vi "stations.vi"(7 "httpRequestID":u32) -> ()   [LabVIEW 2011]
doc: "This VI is a state machine that can be ran from a Browser."
uses:
  server/database/Users/User Record.ctl
  <vilib>/wsapi/NI_WebServices.lvlib
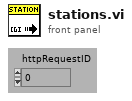
[diagram p1: front panel]
types:
  T1 = typedef "User Record.ctl" = cluster{"ixUser":i32, "sxUsername":string, "sLastName":string, "sFirstName":string, "sEmail":string, "sPassword":string, "tLoginTime":timestamp, "sLoginComputer":string, "fAdministrator":bool, "fRunSequences":bool, "fModifySequences":bool, "fRunScenarios":bool, "fModifyScenarios":bool, "fModifyTemplates":bool, "fModifyUsers":bool, "fModifyStations":bool, "fModifyFields":bool}
  T2 = typedef "Connection Refnum.ctl" = cluster{"Environment Handle":i32, "Connection Handle":i32}
  T3 = typedef "Keyed Array.ctl" = cluster{"keys":string[], "values":string[]}
  T4 = typedef "Station Record.ctl" = cluster{"ixStation":i32, "sxStationId":string, "sIP":string, "fVerified":bool}
  T5 = typedef "Instrument Record.ctl" = cluster{"ixInstrument":i32, "sxInstrumentId":string, "sDriverId":string, "sDriverType":string, "sSerialNumber":string, "tLastCalibration":timestamp, "tCalibrationDue":timestamp, "sConfiguration":string}
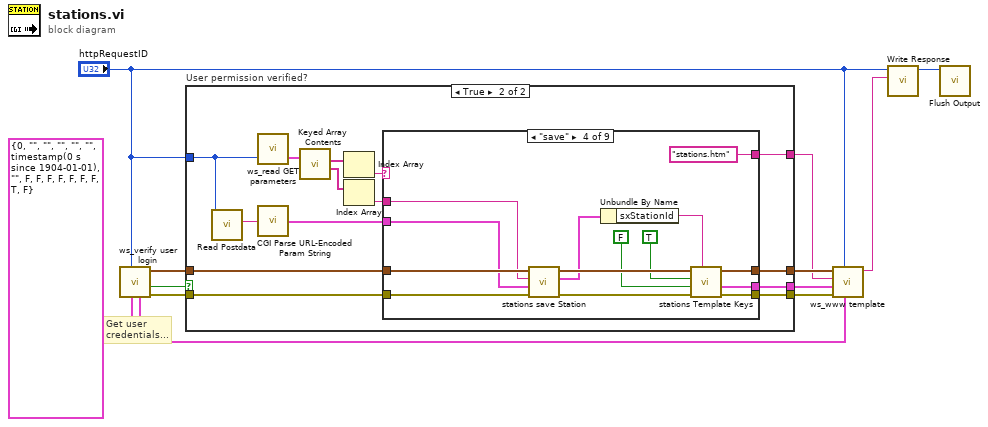
[diagram p0: block diagram]
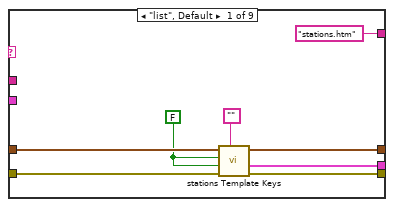
[diagram p3: hidden frame]
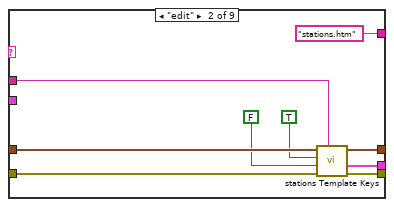
[diagram p4: hidden frame]
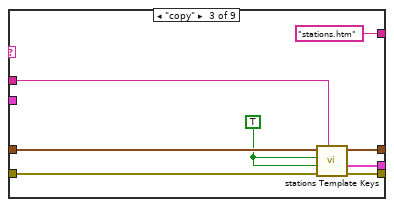
[diagram p5: hidden frame]
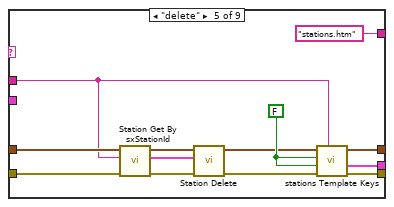
[diagram p6: hidden frame]
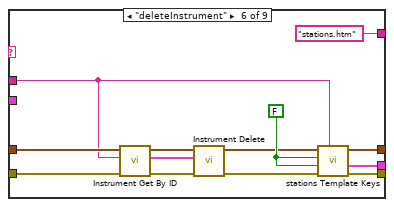
[diagram p7: hidden frame]
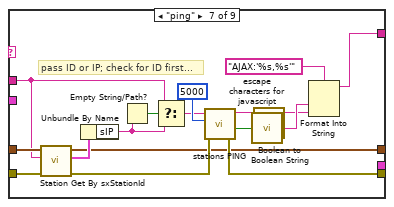
[diagram p8: hidden frame]
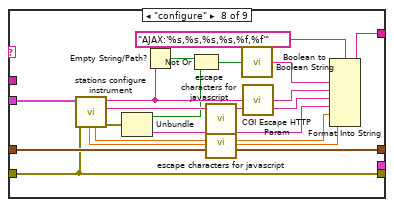
[diagram p9: hidden frame]
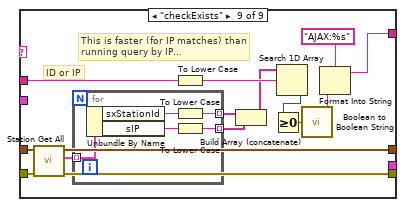
[diagram p10: hidden frame]
diagram:
  # "Get user \ncredentials..."
  n1 = call "ws_verify user login.vi"("Required Permisions"=T1 {"ixUser"=0, "sxUsername"="", "sLastName"="", "sFirstName"="", "sEmail"="", "sPassword"="", "tLoginTime"=timestamp(0 s since 1904-01-01), "sLoginComputer"="", "fAdministrator"=FALSE, "fRunSequences"=FALSE, "fModifySequences"=FALSE, "fRunScenarios"=FALSE, "fModifyScenarios"=FALSE, "fModifyTemplates"=FALSE, "fModifyUsers"=FALSE, "fModifyStations"=TRUE, "fModifyFields"=FALSE} ("User Record"), "httpRequestID"="httpRequestID") -> ("error out"=w6:errorcluster, "User Verified\nand Spartan\nAuthorized?"=w4:bool, "DB Connection Ref"=w5:T2, "User"=w3:T1)  [unwired: 6 in]
  n2 = case "User permission verified?" shown="True" w4 {
    tunnel: w5 -> [w13 w20]
    tunnel: w6 -> [w14 w21]
    tunnel: [w14 w22] -> w11
    tunnel: [_ w19] -> w9
    tunnel: [w13 w17] -> w12
    tunnel: [_ w18] -> w10
    tunnel: "httpRequestID" -> [_ w16]
    frame False {
    }
    frame True {
      n3 = call <vilib>:"Read Postdata.vi"("httpRequestID"=w16) -> ("postdata"=w15:string)  [unwired: 8 in, 2 out]
      n4 = call "ws_read GET parameters.vi"("httpRequestID"=w16) -> ("GET query params"=w23:T3)  [unwired: 2 in]
      n5 = call <vilib>:"CGI Parse URL-Encoded Param String.vi"("url-encoded param string"=w15) -> ("params"=w25:T3)
      n6 = call <vilib>:"Keyed Array Contents.vi"("array in"=w23) -> ("values"=w24:string[], "keys"=w26:string[])  [unwired: 4 in, 1 out]
      n7 = Index Array(array=w26) -> (element=w28:string)  [unwired: 1 in]
      n8 = Index Array(array=w24) -> (element=w27:string)  [unwired: 1 in]
      n9 = case shown="\"save\"" w28 {
        tunnel: w21 -> [w32 w40 w48 w62 w71 w85 w109 w119 w139]
        tunnel: w27 -> [_ w39 w47 w58 w68 w81 w95 _ w134]
        tunnel: [w34 w43 w51 w65 w78 w91 w107 w119 w138] -> w22
        tunnel: w20 -> [w31 w41 w49 w63 w72 w86 w110 w128 w141]
        tunnel: [w35 w44 w52 w66 w79 w92 w105 w128 w140] -> w17
        tunnel: w25 -> [_ _ _ w59 _ _ _ w123 _]
        tunnel: ["stations.htm" ("Template (\"\")") "stations.htm" ("Template (\"\")") "stations.htm" ("Template (\"\")") "stations.htm" ("Template (\"\")") "stations.htm" ("Template (\"\")") "stations.htm" ("Template (\"\")") w104 w113 w142] -> w19
        tunnel: [w33 w42 w50 w64 w77 w90 _ _ _] -> w18
        frame "list", Default {
          w30 = FALSE
          n10 = call "stations Template Keys.vi"("Station ID (\"\")"="", "error in (no error)"=w32, "Copy? (f)"=w30, "Edit? (f)"=w30, "Connection Refnum"=w31) -> ("error out"=w34:errorcluster, "Template Keys"=w33:T3, "Connection Refnum"=w35:T2)  [unwired: 1 in, 3 out]
        }
        frame "edit" {
          n11 = call "stations Template Keys.vi"("Station ID (\"\")"=w39, "error in (no error)"=w40, "Copy? (f)"=FALSE, "Edit? (f)"=TRUE, "Connection Refnum"=w41) -> ("error out"=w43:errorcluster, "Template Keys"=w42:T3, "Connection Refnum"=w44:T2)  [unwired: 1 in, 3 out]
        }
        frame "copy" {
          w46 = TRUE
          n12 = call "stations Template Keys.vi"("Station ID (\"\")"=w47, "error in (no error)"=w48, "Copy? (f)"=w46, "Edit? (f)"=w46, "Connection Refnum"=w49) -> ("error out"=w51:errorcluster, "Template Keys"=w50:T3, "Connection Refnum"=w52:T2)  [unwired: 1 in, 3 out]
        }
        frame "save" {
          n13 = call "stations save Station.vi"("error in (no error)"=w62, "Post Data (empty)"=w59, "Station ID (\"\")"=w58, "Connection Refnum"=w63) -> ("error out"=w61:errorcluster, "Station Record"=w55:T4, "dup Connection Refnum"=w60:T2)  [unwired: 2 in, 3 out]
          n14 = Unbundle By Name(w55) -> ("sxStationId"=w54:string)
          n15 = call "stations Template Keys.vi"("Station ID (\"\")"=w54, "error in (no error)"=w61, "Copy? (f)"=FALSE, "Edit? (f)"=TRUE, "Connection Refnum"=w60) -> ("error out"=w65:errorcluster, "Template Keys"=w64:T3, "Connection Refnum"=w66:T2)  [unwired: 1 in, 3 out]
        }
        frame "delete" {
          w76 = FALSE
          n16 = call "Station Get By sxStationId.vi"("error in (no error)"=w71, "sxStationId (\"\")"=w68, "Connection Refnum"=w72) -> ("error out"=w73:errorcluster, "Station Record"=w75:T4, "Connection Refnum"=w74:T2)  [unwired: 6 out]
          n17 = call "Station Delete.vi"("error in (no error)"=w73, "TestStation Record"=w75, "Connection Refnum"=w74) -> ("error out"=w70:errorcluster, "Connection Refnum"=w69:T2)  [unwired: 7 out]
          n18 = call "stations Template Keys.vi"("Station ID (\"\")"=w68, "error in (no error)"=w70, "Copy? (f)"=w76, "Edit? (f)"=w76, "Connection Refnum"=w69) -> ("error out"=w78:errorcluster, "Template Keys"=w77:T3, "Connection Refnum"=w79:T2)  [unwired: 1 in, 3 out]
        }
        frame "deleteInstrument" {
          w89 = FALSE
          n19 = call "Instrument Get By ID.vi"("error in (no error)"=w85, "sxInstrumentId (\"\")"=w81, "Connection Refnum"=w86) -> ("error out"=w87:errorcluster, "Instrument Record"=w82:T5, "Connection Refnum"=w88:T2)  [unwired: 6 out]
          n20 = call "Instrument Delete.vi"("error in (no error)"=w87, "Instrument Record"=w82, "Connection Refnum"=w88) -> ("error out"=w84:errorcluster, "Connection Refnum"=w83:T2)  [unwired: 7 out]
          n21 = call "stations Template Keys.vi"("Station ID (\"\")"=w81, "error in (no error)"=w84, "Copy? (f)"=w89, "Edit? (f)"=w89, "Connection Refnum"=w83) -> ("error out"=w91:errorcluster, "Template Keys"=w90:T3, "Connection Refnum"=w92:T2)  [unwired: 1 in, 3 out]
        }
        frame "ping" {
          # "pass ID or IP; check for ID first..."
          n22 = call "Station Get By sxStationId.vi"("error in (no error)"=w109, "sxStationId (\"\")"=w95, "Connection Refnum"=w110) -> ("error out"=w108:errorcluster, "Station Record"=w106:T4, "Connection Refnum"=w105:T2)  [unwired: 6 out]
          n23 = Unbundle By Name(w106) -> ("sIP"=w97:string)
          n24 = Empty String/Path?(string/path=w97) -> (empty?=w98:bool)
          n25 = Select(t=w95, s=w98, f=w97) -> (s? t:f=w96:string)
          n26 = call "stations PING.vi"("error in (no error)"=w108, "Ping Timeout (ms)"=5000, "IP Address"=w96) -> ("error out"=w107:errorcluster, "Valid Test Station?"=w102:bool, "PING Response"=w100:string)  [unwired: 3 out]
          n27 = call "Boolean to Boolean String.vi"("Boolean"=w102) -> ("Boolean string"=w101:string)  [unwired: 1 in]
          n28 = call "escape characters for javascript.vi"("String (\"\")"=w100) -> ("escaped String"=w94:string)  [unwired: 4 out]
          n29 = Format Into String(format string="AJAX:'%s,%s'", w101, w94) -> (resulting string=w104:string)  [unwired: 2 in, 1 out]
        }
        frame "configure" {
          n30 = call "stations configure instrument.vi"("error in (no error)"=w119, "POST (empty)"=w123) -> ("error out"=w121:errorcluster, "Serial Number"=w124:string, "Configuration"=w125:string, "LastCal"=w112:dbl, "CalDue"=w111:dbl)  [unwired: 1 in, 4 out]
          n31 = Unbundle(w121) -> ("status"=w117:bool, "source"=w120:string)  [unwired: 1 out]
          n32 = Empty String/Path?(string/path=w125) -> (empty?=w116:bool)
          n33 = Not Or(1:w117, 2:w116) -> (0:w118:bool)
          n34 = call "escape characters for javascript.vi"("String (\"\")"=w124) -> ("escaped String"=w115:string)  [unwired: 4 out]
          n35 = call "escape characters for javascript.vi"("String (\"\")"=w120) -> ("escaped String"=w114:string)  [unwired: 4 out]
          n36 = call "Boolean to Boolean String.vi"("Boolean"=w118) -> ("Boolean string"=w126:string)  [unwired: 1 in]
          n37 = call <vilib>:"CGI Escape HTTP Param.vi"("string"=w125) -> ("url-encoded string"=w122:string)
          n38 = Format Into String(format string="AJAX:'%s,%s,%s,%s,%f,%f'", w126, w122, w115, w114, w112, w111) -> (resulting string=w113:string)  [unwired: 2 in, 1 out]
        }
        frame "checkExists" {
          # "ID or IP"
          # "This is faster (for IP matches) than\nrunning query by IP..."
          n39 = call "Station Get All.vi"("error in (no error)"=w139, "Connection Refnum"=w141) -> ("error out"=w138:errorcluster, "Station Records"=w137:T4[], "Connection Refnum"=w140:T2)  [unwired: 2 in, 5 out]
          n40 = for {
            tunnel: w137 -> [w148] mode=indexing
            tunnel: [w145] -> w136 mode=indexing
            tunnel: [w144] -> w135 mode=indexing
            n41 = Unbundle By Name(w148) -> ("sxStationId"=w147:string, "sIP"=w146:string)
            n42 = To Lower Case(string=w147) -> (all lower case string=w145:string)
            n43 = To Lower Case(string=w146) -> (all lower case string=w144:string)
          }
          n44 = To Lower Case(string=w134) -> (all lower case string=w133:string)
          n45 = Build Array (concatenate)(w136, w135) -> (w132:string[])
          n46 = Search 1D Array(1D array=w132, element=w133) -> (index of element=w130:i32)  [unwired: 1 out]
          n47 = Greater Or Equal To 0?(x=w130) -> (x >= 0?=w129:bool)
          n48 = call "Boolean to Boolean String.vi"("Boolean"=w129) -> ("Boolean string"=w131:string)  [unwired: 1 in]
          n49 = Format Into String(format string="AJAX:%s", w131) -> (resulting string=w142:string)  [unwired: 2 in, 1 out]
        }
      }
    }
  }
  n50 = call "ws_www template.vi"("User"=w3, "httpRequestID"="httpRequestID", "error in (no error)"=w11, "Template Keys (empty)"=w10, "Template (\"\")"=w9, "DB Connection Ref"=w12) -> ("HTTP Template Content"=w8:string)  [unwired: 5 in]
  n51 = call <vilib>:"Write Response.vi"("response string"=w8, "httpRequestID"="httpRequestID") -> ("httpRequestID out"=w7:u32)  [unwired: 8 in, 1 out]
  n52 = call <vilib>:"Flush Output.vi"("httpRequestID"=w7) -> ()  [unwired: 9 in, 2 out]
